vi "BuildErrorMessages.vi"(9 "error in":errorcluster, 10 "ErrorCase":string, 11 "VI Name":string) -> (1 "error out (no error)":errorcluster, 2 "ErrorMessage":string, 5 "call chain":string[](array[string]))   [LabVIEW 2021]
doc: "组建错误信息，\n蒋松\njiangsong@outlook.com\n20140430\n\nDataTime:20151014 10:52:12\nModel:Finance.lvlib:ProjectForecast.lvlib:ProjectForecast.lvclass:Select_Build Work Order 2D Data.vi\nCase:Search: ErrorHandle\nCode:6000\nSource:List Folder in Station.lvclass:CheckStationSharedFolderPathExist.vi->Station1.vi->TopVI.vi<APPEND>\n\\\\192.168.200.250\\d\\13 Engineering\\John Jiang\\Station1"
panel:
  # "DataTime:20151014 10:52:12\nModel:Finance.lvlib:ProjectForecast.lvlib:ProjectForecast.lvclass:Select_Build Work Order 2D Data.vi\nCase:Search: ErrorHandle\nCode:6000\nSource:List Folder in Station.lvclass:CheckStationSharedFolderPathExist.vi->Station1.vi->TopVI.vi<APPEND>\n\\\\192.168.200.250\\d\\13 Engineering\\John Jiang\\Station1"
  # "DateTime---:20200320 14:42:26\nModell-----:GetStationResults.lvlib:GetStationResults.lvclass:Parsing Results String.vi\nCase-------:131234\nCode-------:2345234\nSource-----:In Place Element Structure in Actor Framework.lvlib:Message Priority Queue.lvclass:Priority Enqueue.vi:2960001-\n>GetStationResults.lvlib:Save Data To DB Msg.lvclass:Send Save Data To DB.vi->GetStationResults.lvlib:GetStationResults.lvclass:Parsing Results String.vi"
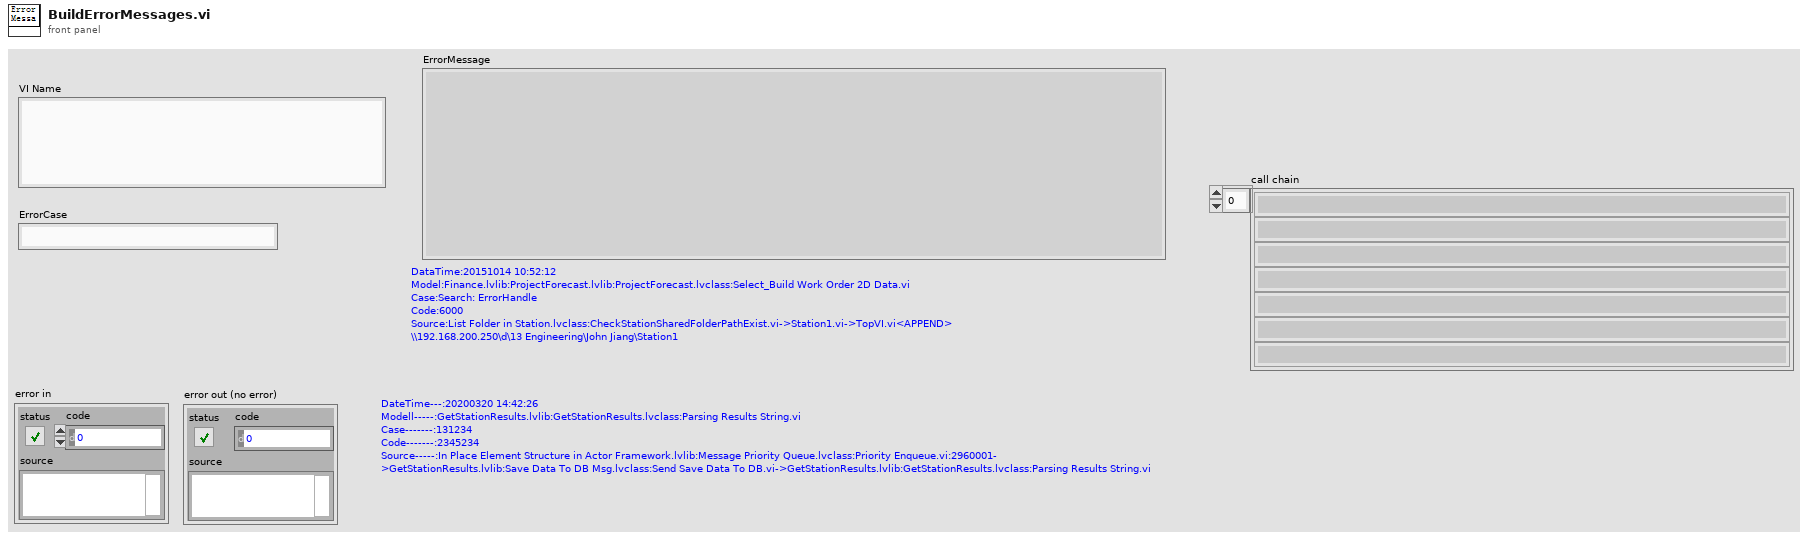
[diagram p1: front panel]
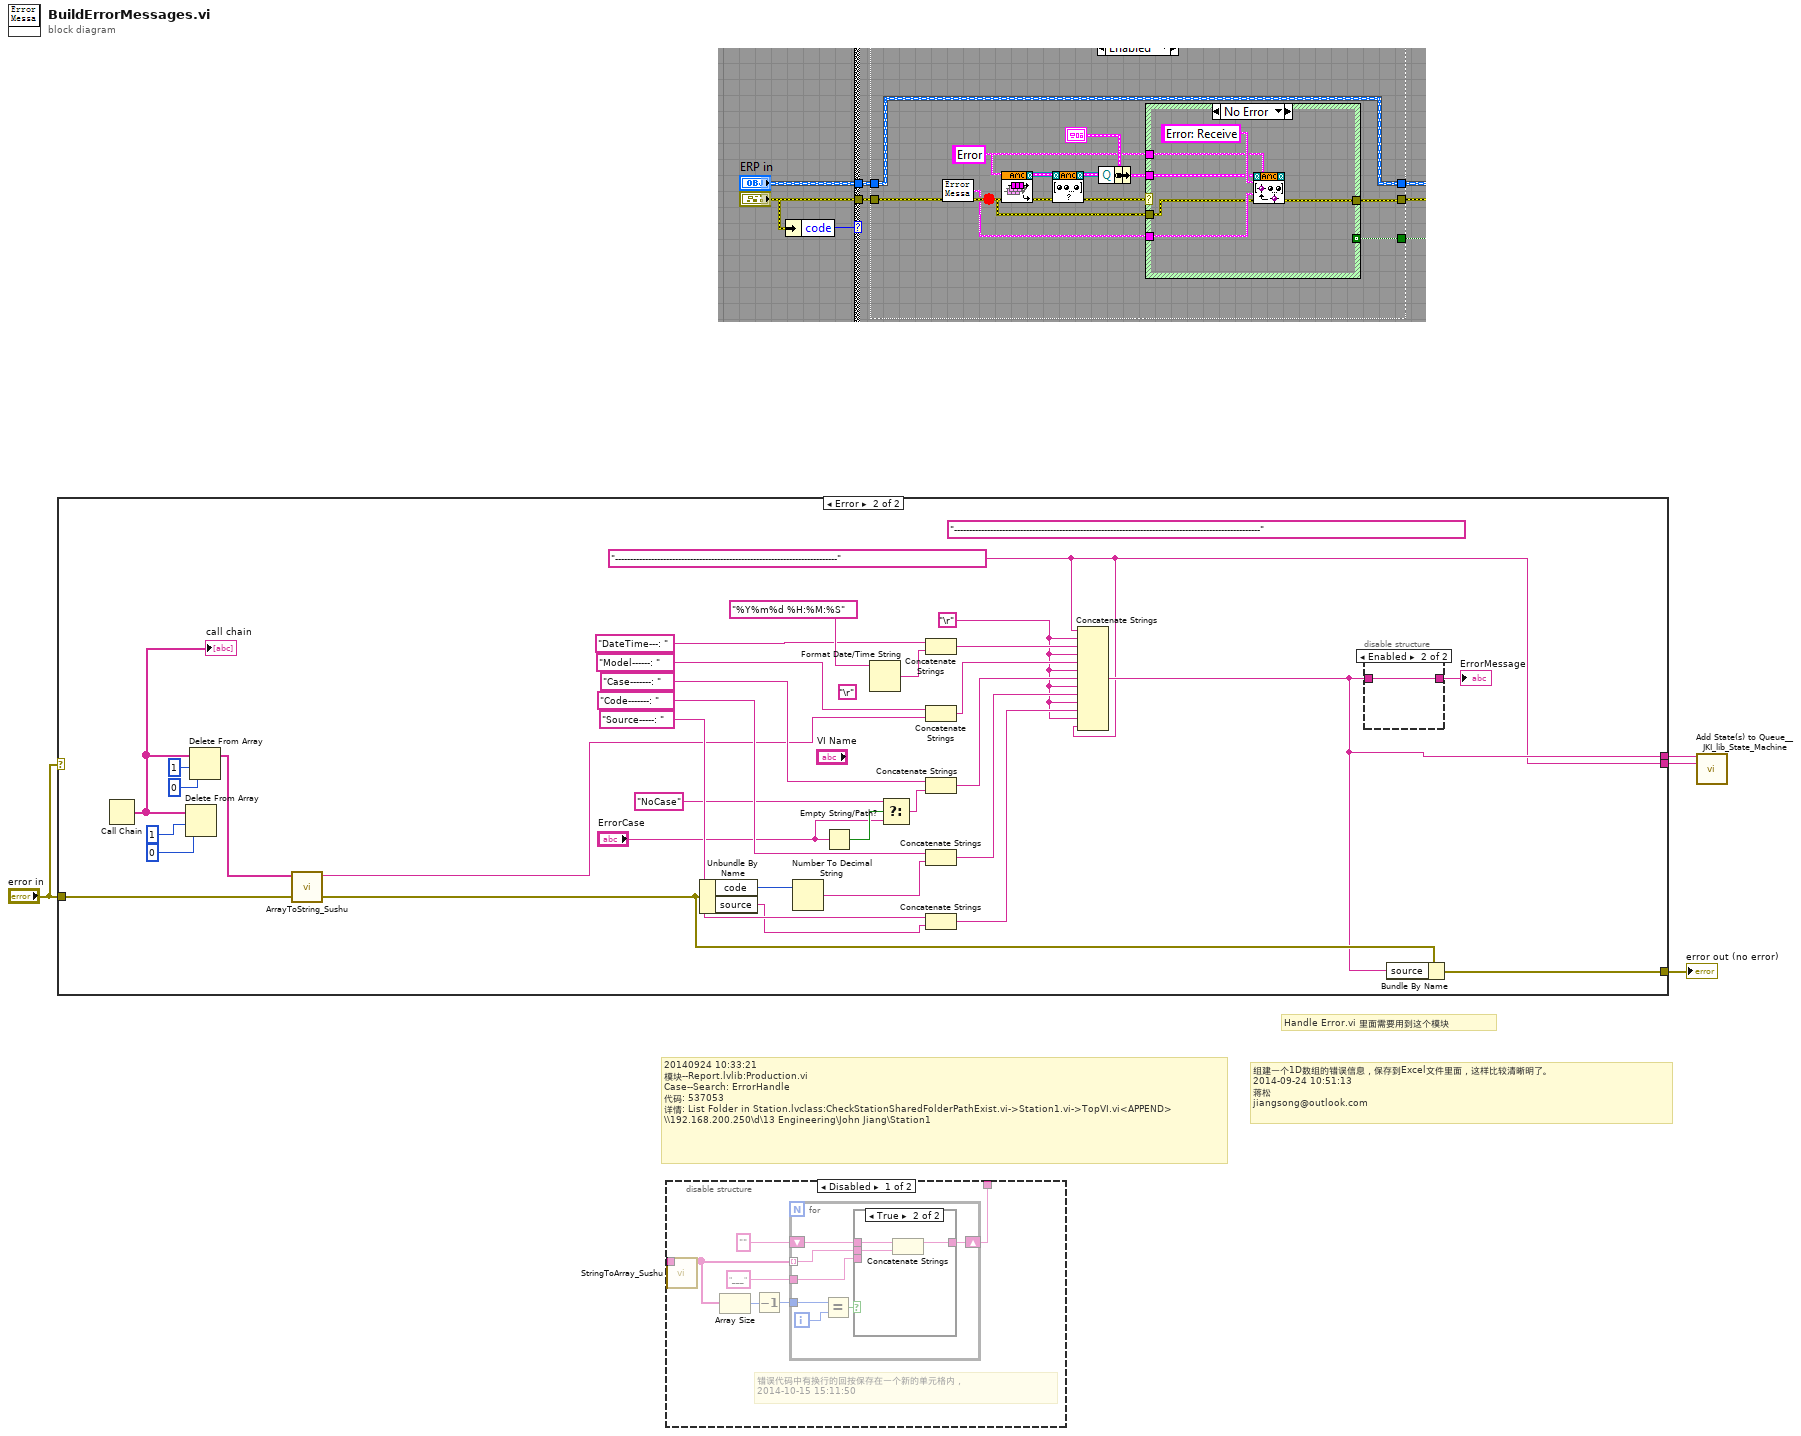
[diagram p0: block diagram]
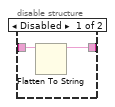
[diagram p3: hidden frame]
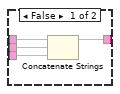
[diagram p4: hidden frame]
diagram:
  # "Handle Error.vi 里面需要用到这个模块"
  # "组建一个1D数组的错误信息，保存到Excel文件里面，这样比较清晰明了。\n2014-09-24 10:51:13\n蒋松\njiangsong@outlook.com"
  # "20140924 10:33:21\n模块--Report.lvlib:Production.vi\nCase--Search: ErrorHandle\n代码: 537053\n详情: List Folder in Station.lvclass:CheckStationSharedFolderPathExist.vi->Station1.vi->TopVI.vi<APPEND>\n\\\\192.168.200.250\\d\\13 Engineering\\John Jiang\\Station1"
  n1 = case shown="Error" "error in" {
    tunnel: "error in" -> [w5 w21]
    tunnel: [w5 w20] -> w4
    tunnel: [_ w19] -> w3
    tunnel: [_ w10] -> w2
    frame No Error {
    }
    frame Error {
      (unwired) "\r"
      (unwired) "------------------------------------------------------------------------------------------------------" ("State(s) in (\"\")")
      w10 = "--------------------------------------------------------------------------" ("State(s) in (\"\")")
      w11 = "\r"
      n2 = Call Chain() -> (call chain=w9:string[])
      "call chain" <- w9
      n3 = Delete From Array(array=w9, length=1, index=0) -> ()  [unwired: 2 out]
      n4 = Delete From Array(array=w9, length=1, index=0) -> (array with subset deleted=w6:string[])  [unwired: 1 out]
      n5 = call <userlib>:"ArrayToString_Sushu.vi"("Array"=w6) -> ("String"=w12:string)  [unwired: 10 in]
      n6 = Unbundle By Name(w21) -> ("code"=w36:i32, "source"=w22:string)
      n7 = Number To Decimal String(number=w36) -> (decimal integer string=w26:string)  [unwired: 1 in]
      n8 = Empty String/Path?(string/path="ErrorCase") -> (empty?=w18:bool)
      n9 = Format Date/Time String(time format string (%c)="%Y%m%d %H:%M:%S") -> (date/time string=w32:string)  [unwired: 2 in]
      n10 = Select(t="NoCase", s=w18, f="ErrorCase") -> (s? t:f=w16:string)
      n11 = Concatenate Strings("DateTime---: " ("string"), w32) -> (w31:string)
      n12 = Concatenate Strings("Model------: " ("string"), w12) -> (w30:string)
      n13 = Concatenate Strings("Case-------: " ("string"), w16) -> (w28:string)
      n14 = Concatenate Strings("Code-------: " ("string"), w26) -> (w24:string)
      n15 = Concatenate Strings("Source-----: " ("string"), w22) -> (w23:string)
      n16 = Concatenate Strings(w10, w11, w31, w11, w30, w11, w28, w11, w24, w11, w23, w11, w10) -> (w19:string)
      n17 = disable-structure shown="Enabled" {
        disable-tunnel: [w39 w40] -> w35
        disable-tunnel: w19 -> [w38 w40]
        frame Disabled {
          n18 = Flatten To String(anything=w38) -> (data string=w39:string)  [unwired: 3 in, 2 out]
        }
        frame Enabled {
        }
      }
      "ErrorMessage" <- w35
      n19 = Bundle By Name(cluster=w21, "source"=w19) -> (w20:errorcluster)
    }
  }
  "error out (no error)" <- w4
  n20 = disable-structure shown="Disabled" {
    disable-tunnel: _ -> [w42 _]
    disable-tunnel: [w41 _] -> _
    frame Disabled {
      # "错误代码中有换行的回按保存在一个新的单元格内，\n2014-10-15 15:11:50"
      n21 = call <userlib>:"StringToArray_Sushu.vi"("State Queue"=w42) -> ("Array"=w45:string[])  [unwired: 7 in, 3 out]
      n22 = Array Size(array=w45) -> (size(s)=w46:i32)
      n23 = Decrement(x=w46) -> (x-1=w47:i32)
      n24 = for {
        shift-right: [w53] -> w41
        shift-left: "" ("trimmed string") -> [w54]
        tunnel: w45 -> [w52] mode=indexing
        tunnel: "___" ("string") -> [w51]
        tunnel: w47 -> [w49]
        i -> [w50]
        n25 = Equal?(x=w49, y=w50) -> (x = y?=w48:bool)
        n26 = case shown="True" w48 {
          tunnel: w54 -> [w58 w61]
          tunnel: [w57 w60] -> w53
          tunnel: w52 -> [w56 w59]
          tunnel: w51 -> [w55 _]
          frame False {
            n27 = Concatenate Strings(w58, w56, w55) -> (w57:string)
          }
          frame True {
            n28 = Concatenate Strings(w61, w59) -> (w60:string)
          }
        }
      }
    }
    frame Enabled {
    }
  }
  n29 = call <vilib>:"Add State(s) to Queue__JKI_lib_State_Machine.vi"("State(s) in Front (\"\")"=w3, "State(s) in (\"\")"=w2) -> ()  [unwired: 13 in, 1 out]
